vi "HEWH Gather Test Data.vi"(0 "MW100":refnum<visa-resource-name>="MW100", 1 "Core HEWH Data Station A":T2={"Scan Rate Adjust"=0.0, "Draw Count"=0, "Test Patten Setup"={"Total Gallons Schedule"=[], "PRAT/RLT Sequence"=[{"Sequence #"=1.0, "Cycles"=35, "Mode Setting"="", "Flow Rate (GPM)"=0.0, "Temperature (F)"=0.0, "Reset Timer"=FALSE, "Use Temp Decline Method"=FALSE, "Terminate Condition"=enum."C1-Terminate Draw @ Gallon Mark", "Condition Value #1"=0.0, "UE"=FALSE, "LE"=FALSE, "Comp"=FALSE, "Fan"=FALSE, "Test End Time (Sec)"=0.0, "Purge Until Cutout"=FALSE, "Start Conditions"=enum."Heat Source Cutout", "Condition Value #2"=0.0, "Remove Power"=FALSE, "Time"=0.0, "Check Special Cond."=enum."SC1-Do Nothing", "Condition#"=enum."C1", "Draw Flags"=enum."N/A", "Data Processing Delay (FHD 15sec, UEF 5 Sec)"=0.0, "Test Complete"=FALSE}, {"Sequence #"=2.0, "Cycles"=15, "Mode Setting"="", "Flow Rate (GPM)"=0.0, "Temperature (F)"=0.0, "Reset Timer"=FALSE, "Use Temp Decline Method"=FALSE, "Terminate Condition"=enum."C1-Terminate Draw @ Gallon Mark", "Condition Value #1"=0.0, "UE"=FALSE, "LE"=FALSE, "Comp"=FALSE, "Fan"=FALSE, "Test End Time (Sec)"=0.0, "Purge Until Cutout"=FALSE, "Start Conditions"=enum."Heat Source Cutout", "Condition Value #2"=0.0, "Remove Power"=FALSE, "Time"=0.0, "Check Special Cond."=enum."SC1-Do Nothing", "Condition#"=enum."C1", "Draw Flags"=enum."N/A", "Data Processing Delay (FHD 15sec, UEF 5 Sec)"=0.0, "Test Complete"=FALSE}, {"Sequence #"=3.0, "Cycles"=35, "Mode Setting"="", "Flow Rate (GPM)"=0.0, "Temperature (F)"=0.0, "Reset Timer"=FALSE, "Use Temp Decline Method"=FALSE, "Terminate Condition"=enum."C1-Terminate Draw @ Gallon Mark", "Condition Value #1"=0.0, "UE"=FALSE, "LE"=FALSE, "Comp"=FALSE, "Fan"=FALSE, "Test End Time (Sec)"=0.0, "Purge Until Cutout"=FALSE, "Start Conditions"=enum."Heat Source Cutout", "Condition Value #2"=0.0, "Remove Power"=FALSE, "Time"=0.0, "Check Special Cond."=enum."SC1-Do Nothing", "Condition#"=enum."C1", "Draw Flags"=enum."N/A", "Data Processing Delay (FHD 15sec, UEF 5 Sec)"=0.0, "Test Complete"=FALSE}, {"Sequence #"=4.0, "Cycles"=15, "Mode Setting"="", "Flow Rate (GPM)"=0.0, "Temperature (F)"=0.0, "Reset Timer"=FALSE, "Use Temp Decline Method"=FALSE, "Terminate Condition"=enum."C1-Terminate Draw @ Gallon Mark", "Condition Value #1"=0.0, "UE"=FALSE, "LE"=FALSE, "Comp"=FALSE, "Fan"=FALSE, "Test End Time (Sec)"=0.0, "Purge Until Cutout"=FALSE, "Start Conditions"=enum."Heat Source Cutout", "Condition Value #2"=0.0, "Remove Power"=FALSE, "Time"=0.0, "Check Special Cond."=enum."SC1-Do Nothing", "Condition#"=enum."C1", "Draw Flags"=enum."N/A", "Data Processing Delay (FHD 15sec, UEF 5 Sec)"=0.0, "Test Complete"=FALSE}, {"Sequence #"=5.0, "Cycles"=35, "Mode Setting"="", "Flow Rate (GPM)"=0.0, "Temperature (F)"=0.0, "Reset Timer"=FALSE, "Use Temp Decline Method"=FALSE, "Terminate Condition"=enum."C1-Terminate Draw @ Gallon Mark", "Condition Value #1"=0.0, "UE"=FALSE, "LE"=FALSE, "Comp"=FALSE, "Fan"=FALSE, "Test End Time (Sec)"=0.0, "Purge Until Cutout"=FALSE, "Start Conditions"=enum."Heat Source Cutout", "Condition Value #2"=0.0, "Remove Power"=FALSE, "Time"=0.0, "Check Special Cond."=enum."SC1-Do Nothing", "Condition#"=enum."C1", "Draw Flags"=enum."N/A", "Data Processing Delay (FHD 15sec, UEF 5 Sec)"=0.0, "Test Complete"=FALSE}, {"Sequence #"=6.0, "Cycles"=15, "Mode Setting"="", "Flow Rate (GPM)"=0.0, "Temperature (F)"=0.0, "Reset Timer"=FALSE, "Use Temp Decline Method"=FALSE, "Terminate Condition"=enum."C1-Terminate Draw @ Gallon Mark", "Condition Value #1"=0.0, "UE"=FALSE, "LE"=FALSE, "Comp"=FALSE, "Fan"=FALSE, "Test End Time (Sec)"=0.0, "Purge Until Cutout"=FALSE, "Start Conditions"=enum."Heat Source Cutout", "Condition Value #2"=0.0, "Remove Power"=FALSE, "Time"=0.0, "Check Special Cond."=enum."SC1-Do Nothing", "Condition#"=enum."C1", "Draw Flags"=enum."N/A", "Data Processing Delay (FHD 15sec, UEF 5 Sec)"=0.0, "Test Complete"=FALSE}, {"Sequence #"=7.0, "Cycles"=35, "Mode Setting"="", "Flow Rate (GPM)"=0.0, "Temperature (F)"=0.0, "Reset Timer"=FALSE, "Use Temp Decline Method"=FALSE, "Terminate Condition"=enum."C1-Terminate Draw @ Gallon Mark", "Condition Value #1"=0.0, "UE"=FALSE, "LE"=FALSE, "Comp"=FALSE, "Fan"=FALSE, "Test End Time (Sec)"=0.0, "Purge Until Cutout"=FALSE, "Start Conditions"=enum."Heat Source Cutout", "Condition Value #2"=0.0, "Remove Power"=FALSE, "Time"=0.0, "Check Special Cond."=enum."SC1-Do Nothing", "Condition#"=enum."C1", "Draw Flags"=enum."N/A", "Data Processing Delay (FHD 15sec, UEF 5 Sec)"=0.0, "Test Complete"=FALSE}, {"Sequence #"=8.0, "Cycles"=15, "Mode Setting"="", "Flow Rate (GPM)"=0.0, "Temperature (F)"=0.0, "Reset Timer"=FALSE, "Use Temp Decline Method"=FALSE, "Terminate Condition"=enum."C1-Terminate Draw @ Gallon Mark", "Condition Value #1"=0.0, "UE"=FALSE, "LE"=FALSE, "Comp"=FALSE, "Fan"=FALSE, "Test End Time (Sec)"=0.0, "Purge Until Cutout"=FALSE, "Start Conditions"=enum."Heat Source Cutout", "Condition Value #2"=0.0, "Remove Power"=FALSE, "Time"=0.0, "Check Special Cond."=enum."SC1-Do Nothing", "Condition#"=enum."C1", "Draw Flags"=enum."N/A", "Data Processing Delay (FHD 15sec, UEF 5 Sec)"=0.0, "Test Complete"=FALSE}], "Current Sequence Index"=0}, "HEWH Specific DAQ"={"HEWH Data"={"HEWH Standard"={"Voltage (Volts)"=0.0, "Current (Amps)"=0.0, "Power (Watts)"=0.0, "WattHours (Wh)"=0.0, "TC Tree (AVG)"=0.0, "Flow Rate (GPM)"=0.0, "Gallons (Gal)"=0.0, "RTD Out (Deg F)"=0.0, "RTD In (Deg F)"=0.0, "RTD Amb (Deg F)"=0.0, "TC Down"=0.0, "UE Event Lead"=0, "LE Event Lead"=0, "TC Tree Array"=[]}, "PRAT"={"Power (Watts) A"=4192.0, "Power (Watts) B"=4192.0, "Power (Watts) C"=4192.0, "Power (Watts) D"=4192.0, "TC1"=0.0, "TC2"=0.0, "TC3"=0.0, "TC4"=0.0, "WattHours (Wh) A"=4192.0, "WattHours (Wh) B"=4192.0, "WattHours (Wh) C"=4192.0, "WattHours (Wh) D"=4192.0, "Ambient"=0.0, "Extra Temp"=0.0}, "Additional Power Data"={"Vthd"=236.2, "Frequency (Hz)"=236.2, "Apparent Power (VA)"=236.2, "Power Factor"=236.2, "Current Crest Factor"=236.2, "Voltage Crest Factor"=236.2, "Integration Time (sec)"=236.2}}, "Flow Valve % Open"=0.0, "Power State"={"UE"=FALSE, "LE"=FALSE, "COMP"=FALSE, "FANS"=FALSE}, "Power Analyzer"=enum."APLUS", "Flow Valve uA Output"=0, "Gallons Start (Gal)"=0.0}, "Test Output Data"={"PreDraw Data Table"=[], "Data Table"=[], "MW100 TC Headers"=[]}, "Calc and Calibration"={"Mean SD Var Max Min Array"=[], "Draw Statistics (DBL)"=[], "Calibration Coefficients DBL"=[], "Start Gallons"=0.0, "Starting Temp Decline"=0.0, "K-Factor (Intellifaucet)"=0.0, "All Draw Stats"=[], "RTD Terminate Value"=0.0}, "Current Draw Time"=0.0, "LV Program"=enum."HEWH", "Station ID"=enum."A", "Current Cond"=enum."N/A", "Test Complete"=FALSE} {"Test Patten Setup"."PRAT/RLT Sequence"."Time" format="%<%H:%M:%S>t"; "Test Patten Setup"."Total Gallons Schedule" format="%.2f"}, 2 "GEA2?":bool, 4 "Yokogawa WT210":refnum<visa-resource-name>, 5 "error in (no error)":errorcluster, 6 "Laurel IP Address":string, 9 "Draw Count":i32, 11 "Use Emerson 5700?":bool) -> (14 "MW100 Output":refnum<visa-resource-name>, 15 "Core HEWH Data Station A":T2={"Scan Rate Adjust"=0.0, "Draw Count"=0, "Test Patten Setup"={"Total Gallons Schedule"=[], "PRAT/RLT Sequence"=[{"Sequence #"=1.0, "Cycles"=35, "Mode Setting"="", "Flow Rate (GPM)"=0.0, "Temperature (F)"=0.0, "Reset Timer"=FALSE, "Use Temp Decline Method"=FALSE, "Terminate Condition"=enum."C1-Terminate Draw @ Gallon Mark", "Condition Value #1"=0.0, "UE"=FALSE, "LE"=FALSE, "Comp"=FALSE, "Fan"=FALSE, "Test End Time (Sec)"=0.0, "Purge Until Cutout"=FALSE, "Start Conditions"=enum."Heat Source Cutout", "Condition Value #2"=0.0, "Remove Power"=FALSE, "Time"=0.0, "Check Special Cond."=enum."SC1-Do Nothing", "Condition#"=enum."C1", "Draw Flags"=enum."N/A", "Data Processing Delay (FHD 15sec, UEF 5 Sec)"=0.0, "Test Complete"=FALSE}, {"Sequence #"=2.0, "Cycles"=15, "Mode Setting"="", "Flow Rate (GPM)"=0.0, "Temperature (F)"=0.0, "Reset Timer"=FALSE, "Use Temp Decline Method"=FALSE, "Terminate Condition"=enum."C1-Terminate Draw @ Gallon Mark", "Condition Value #1"=0.0, "UE"=FALSE, "LE"=FALSE, "Comp"=FALSE, "Fan"=FALSE, "Test End Time (Sec)"=0.0, "Purge Until Cutout"=FALSE, "Start Conditions"=enum."Heat Source Cutout", "Condition Value #2"=0.0, "Remove Power"=FALSE, "Time"=0.0, "Check Special Cond."=enum."SC1-Do Nothing", "Condition#"=enum."C1", "Draw Flags"=enum."N/A", "Data Processing Delay (FHD 15sec, UEF 5 Sec)"=0.0, "Test Complete"=FALSE}, {"Sequence #"=3.0, "Cycles"=35, "Mode Setting"="", "Flow Rate (GPM)"=0.0, "Temperature (F)"=0.0, "Reset Timer"=FALSE, "Use Temp Decline Method"=FALSE, "Terminate Condition"=enum."C1-Terminate Draw @ Gallon Mark", "Condition Value #1"=0.0, "UE"=FALSE, "LE"=FALSE, "Comp"=FALSE, "Fan"=FALSE, "Test End Time (Sec)"=0.0, "Purge Until Cutout"=FALSE, "Start Conditions"=enum."Heat Source Cutout", "Condition Value #2"=0.0, "Remove Power"=FALSE, "Time"=0.0, "Check Special Cond."=enum."SC1-Do Nothing", "Condition#"=enum."C1", "Draw Flags"=enum."N/A", "Data Processing Delay (FHD 15sec, UEF 5 Sec)"=0.0, "Test Complete"=FALSE}, {"Sequence #"=4.0, "Cycles"=15, "Mode Setting"="", "Flow Rate (GPM)"=0.0, "Temperature (F)"=0.0, "Reset Timer"=FALSE, "Use Temp Decline Method"=FALSE, "Terminate Condition"=enum."C1-Terminate Draw @ Gallon Mark", "Condition Value #1"=0.0, "UE"=FALSE, "LE"=FALSE, "Comp"=FALSE, "Fan"=FALSE, "Test End Time (Sec)"=0.0, "Purge Until Cutout"=FALSE, "Start Conditions"=enum."Heat Source Cutout", "Condition Value #2"=0.0, "Remove Power"=FALSE, "Time"=0.0, "Check Special Cond."=enum."SC1-Do Nothing", "Condition#"=enum."C1", "Draw Flags"=enum."N/A", "Data Processing Delay (FHD 15sec, UEF 5 Sec)"=0.0, "Test Complete"=FALSE}, {"Sequence #"=5.0, "Cycles"=35, "Mode Setting"="", "Flow Rate (GPM)"=0.0, "Temperature (F)"=0.0, "Reset Timer"=FALSE, "Use Temp Decline Method"=FALSE, "Terminate Condition"=enum."C1-Terminate Draw @ Gallon Mark", "Condition Value #1"=0.0, "UE"=FALSE, "LE"=FALSE, "Comp"=FALSE, "Fan"=FALSE, "Test End Time (Sec)"=0.0, "Purge Until Cutout"=FALSE, "Start Conditions"=enum."Heat Source Cutout", "Condition Value #2"=0.0, "Remove Power"=FALSE, "Time"=0.0, "Check Special Cond."=enum."SC1-Do Nothing", "Condition#"=enum."C1", "Draw Flags"=enum."N/A", "Data Processing Delay (FHD 15sec, UEF 5 Sec)"=0.0, "Test Complete"=FALSE}, {"Sequence #"=6.0, "Cycles"=15, "Mode Setting"="", "Flow Rate (GPM)"=0.0, "Temperature (F)"=0.0, "Reset Timer"=FALSE, "Use Temp Decline Method"=FALSE, "Terminate Condition"=enum."C1-Terminate Draw @ Gallon Mark", "Condition Value #1"=0.0, "UE"=FALSE, "LE"=FALSE, "Comp"=FALSE, "Fan"=FALSE, "Test End Time (Sec)"=0.0, "Purge Until Cutout"=FALSE, "Start Conditions"=enum."Heat Source Cutout", "Condition Value #2"=0.0, "Remove Power"=FALSE, "Time"=0.0, "Check Special Cond."=enum."SC1-Do Nothing", "Condition#"=enum."C1", "Draw Flags"=enum."N/A", "Data Processing Delay (FHD 15sec, UEF 5 Sec)"=0.0, "Test Complete"=FALSE}, {"Sequence #"=7.0, "Cycles"=35, "Mode Setting"="", "Flow Rate (GPM)"=0.0, "Temperature (F)"=0.0, "Reset Timer"=FALSE, "Use Temp Decline Method"=FALSE, "Terminate Condition"=enum."C1-Terminate Draw @ Gallon Mark", "Condition Value #1"=0.0, "UE"=FALSE, "LE"=FALSE, "Comp"=FALSE, "Fan"=FALSE, "Test End Time (Sec)"=0.0, "Purge Until Cutout"=FALSE, "Start Conditions"=enum."Heat Source Cutout", "Condition Value #2"=0.0, "Remove Power"=FALSE, "Time"=0.0, "Check Special Cond."=enum."SC1-Do Nothing", "Condition#"=enum."C1", "Draw Flags"=enum."N/A", "Data Processing Delay (FHD 15sec, UEF 5 Sec)"=0.0, "Test Complete"=FALSE}, {"Sequence #"=8.0, "Cycles"=15, "Mode Setting"="", "Flow Rate (GPM)"=0.0, "Temperature (F)"=0.0, "Reset Timer"=FALSE, "Use Temp Decline Method"=FALSE, "Terminate Condition"=enum."C1-Terminate Draw @ Gallon Mark", "Condition Value #1"=0.0, "UE"=FALSE, "LE"=FALSE, "Comp"=FALSE, "Fan"=FALSE, "Test End Time (Sec)"=0.0, "Purge Until Cutout"=FALSE, "Start Conditions"=enum."Heat Source Cutout", "Condition Value #2"=0.0, "Remove Power"=FALSE, "Time"=0.0, "Check Special Cond."=enum."SC1-Do Nothing", "Condition#"=enum."C1", "Draw Flags"=enum."N/A", "Data Processing Delay (FHD 15sec, UEF 5 Sec)"=0.0, "Test Complete"=FALSE}], "Current Sequence Index"=0}, "HEWH Specific DAQ"={"HEWH Data"={"HEWH Standard"={"Voltage (Volts)"=0.0, "Current (Amps)"=0.0, "Power (Watts)"=0.0, "WattHours (Wh)"=0.0, "TC Tree (AVG)"=0.0, "Flow Rate (GPM)"=0.0, "Gallons (Gal)"=0.0, "RTD Out (Deg F)"=0.0, "RTD In (Deg F)"=0.0, "RTD Amb (Deg F)"=0.0, "TC Down"=0.0, "UE Event Lead"=0, "LE Event Lead"=0, "TC Tree Array"=[]}, "PRAT"={"Power (Watts) A"=4192.0, "Power (Watts) B"=4192.0, "Power (Watts) C"=4192.0, "Power (Watts) D"=4192.0, "TC1"=0.0, "TC2"=0.0, "TC3"=0.0, "TC4"=0.0, "WattHours (Wh) A"=4192.0, "WattHours (Wh) B"=4192.0, "WattHours (Wh) C"=4192.0, "WattHours (Wh) D"=4192.0, "Ambient"=0.0, "Extra Temp"=0.0}, "Additional Power Data"={"Vthd"=236.2, "Frequency (Hz)"=236.2, "Apparent Power (VA)"=236.2, "Power Factor"=236.2, "Current Crest Factor"=236.2, "Voltage Crest Factor"=236.2, "Integration Time (sec)"=236.2}}, "Flow Valve % Open"=0.0, "Power State"={"UE"=FALSE, "LE"=FALSE, "COMP"=FALSE, "FANS"=FALSE}, "Power Analyzer"=enum."APLUS", "Flow Valve uA Output"=0, "Gallons Start (Gal)"=0.0}, "Test Output Data"={"PreDraw Data Table"=[], "Data Table"=[], "MW100 TC Headers"=[]}, "Calc and Calibration"={"Mean SD Var Max Min Array"=[], "Draw Statistics (DBL)"=[], "Calibration Coefficients DBL"=[], "Start Gallons"=0.0, "Starting Temp Decline"=0.0, "K-Factor (Intellifaucet)"=0.0, "All Draw Stats"=[], "RTD Terminate Value"=0.0}, "Current Draw Time"=0.0, "LV Program"=enum."HEWH", "Station ID"=enum."A", "Current Cond"=enum."N/A", "Test Complete"=FALSE} {"Test Patten Setup"."PRAT/RLT Sequence"."Time" format="%<%H:%M:%S>t"; "Test Patten Setup"."Total Gallons Schedule" format="%.2f"}, 16 "Display Message":string, 17 "Emerson Flow Meter Data Output":T1, 18 "MW100 Full Data":string[][](array[string]), 19 "error out":errorcluster={"status"=TRUE, "code"=-1073807346, "source"="VISA Read in Gather Test Data.vi"})   [LabVIEW 2016]
uses:
  Type Definitions/HEWH Output Information.ctl
  Type Definitions/HEWH Draw Pattern Setup.ctl
  Type Definitions/PRAT Test.ctl
  Utility/Save File/File Setup (Public)/Type Definition/Save File HEWH Heating Control Mode.ctl
  Support VIs/Draw Water Specific/Type Definitions/Terminate Draw Conditions.ctl
  Type Definitions/HEWH Start Conditions.ctl
  Support VIs/Draw Water Specific/Type Definitions/Check Special Condtions.ctl
  Support VIs/Draw Water Specific/Type Definitions/HEWH Special Condition Check.ctl
  Type Definitions/HEWH Draw Flag ENUM.ctl
  Type Definitions/HEWH Specific DAQ.ctl
  Type Definitions/HEWH Power Data.ctl
  Type Definitions/HEWH Power Elements.ctl
  Utility/Type Definitions/UTILITY Power Analyzer.ctl
  Type Definitions/HEWH Calc and Calibration.ctl
  Utility/Save File/File Setup (Public)/Type Definition/Save File DOE LabView Program.ctl
  MW100/Type Definitions/Station ID Selector.ctl
  Drivers/Emerson 5700 Transmitter/Type Definitions/Emerson 5700 Data.ctl
  Utility/Type Definitions/UTILITY Power Data.ctl
  Drivers/Laurel Meter/Type Definitions/Laurel Serial Commands.ctl
  Type Definitions/HEWH MW100 Data Cluster.ctl
  Utility/Save File/File Setup.lvlib
panel:
  # "Draw Pattern Setup (24 Hour)"
  # "Draw Pattern Setup (24 Hour)"
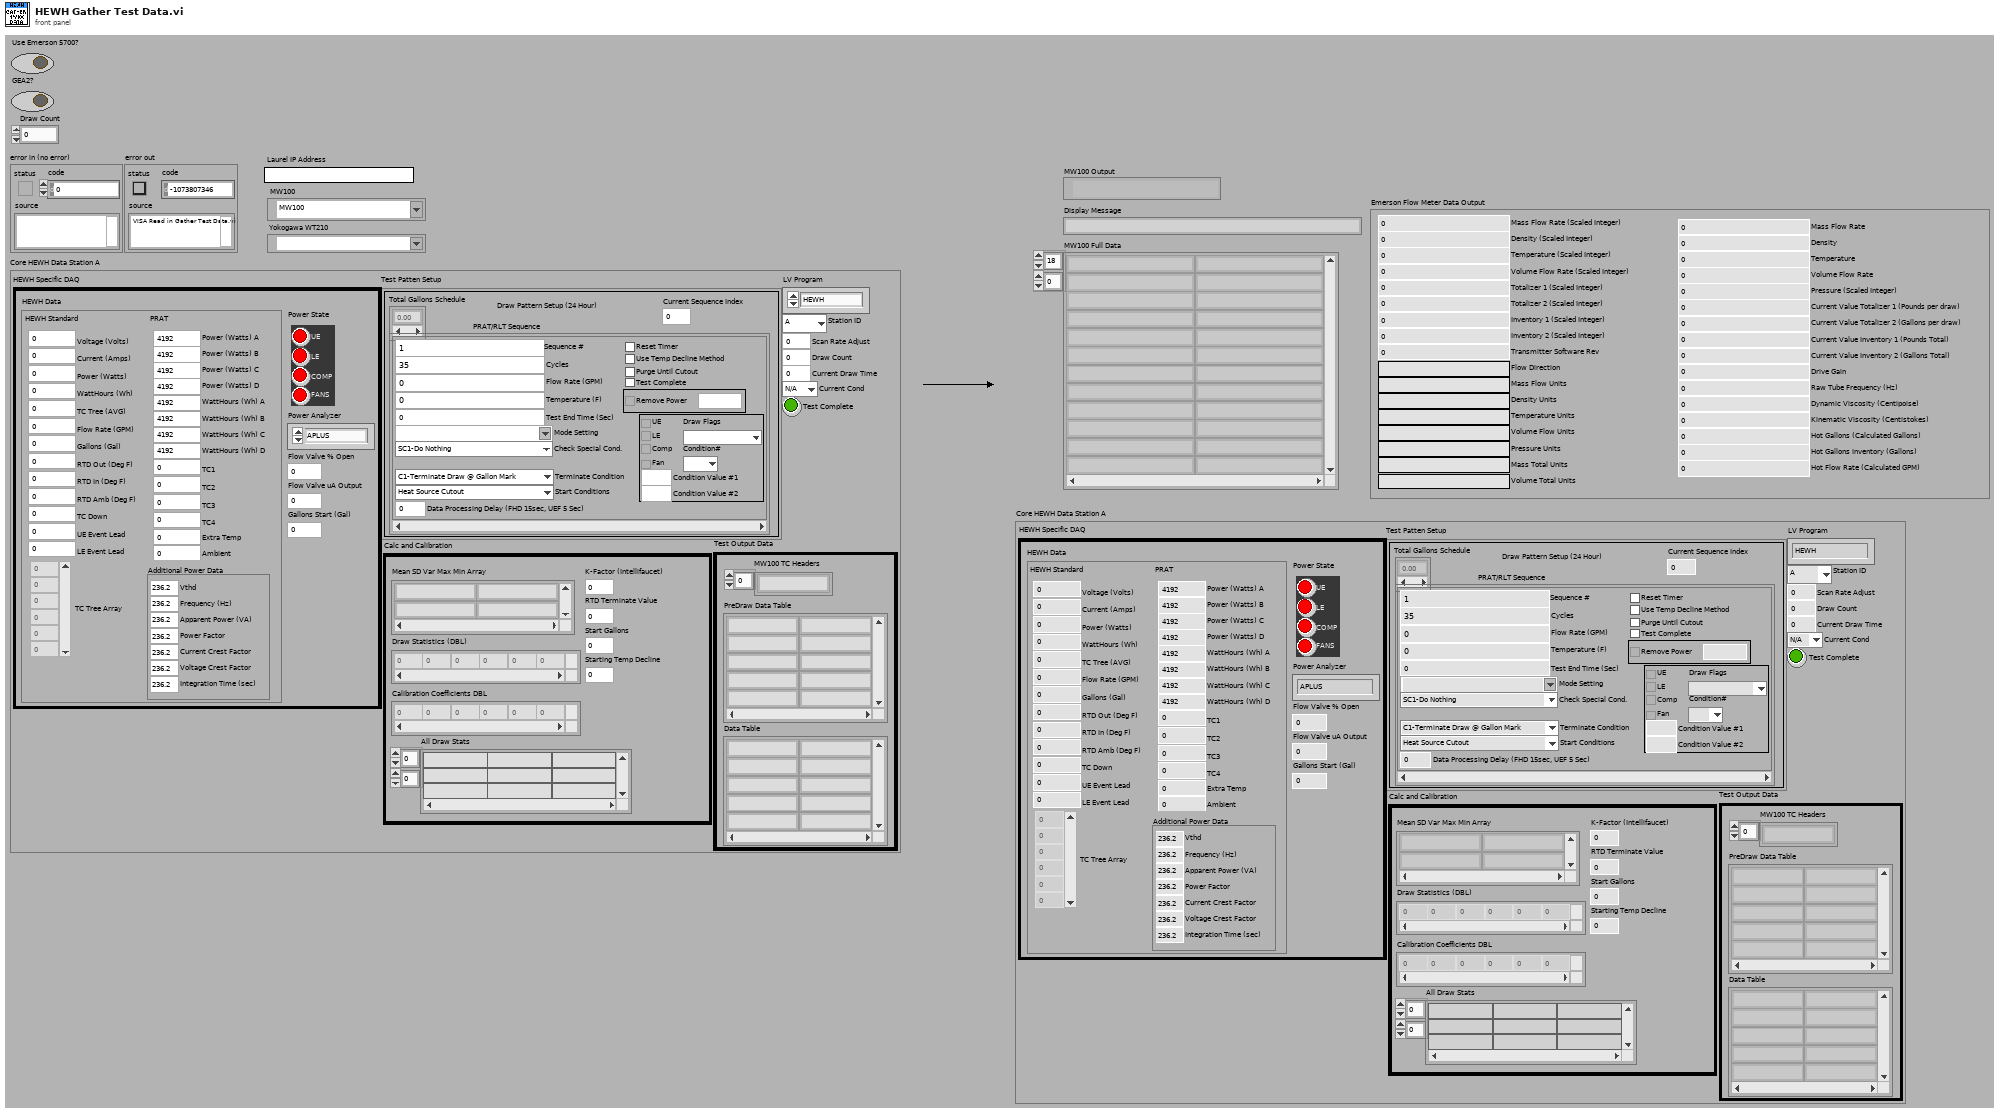
[diagram p1: front panel]
types:
  T1 = typedef "Emerson 5700 Data.ctl" = cluster{"Mass Flow Rate (Scaled Integer)":u16, "Density (Scaled Integer)":u16, "Temperature (Scaled Integer)":u16, "Volume Flow Rate (Scaled Integer)":u16, "Totalizer 1 (Scaled Integer)":u16, "Totalizer 2 (Scaled Integer)":u16, "Transmitter Software Rev":u16, "Flow Direction":string, "Mass Flow Units":string, "Density Units":string, "Temperature Units":string, "Volume Flow Units":string, "Pressure Units":string, "Mass Total Units":string, "Volume Total Units":string, "Inventory 1 (Scaled Integer)":u16, "Inventory 2 (Scaled Integer)":u16, "Mass Flow Rate":dbl, "Density":dbl, "Temperature":dbl, "Volume Flow Rate":dbl, "Pressure (Scaled Integer)":u16, "Current Value Totalizer 1 (Pounds per draw)":dbl, "Current Value Totalizer 2 (Gallons per draw)":dbl, "Current Value Inventory 1 (Pounds Total)":dbl, "Current Value Inventory 2 (Gallons Total)":dbl, "Drive Gain":dbl, "Raw Tube Frequency (Hz)":dbl, "Dynamic Viscosity (Centipoise)":dbl, "Kinematic Viscosity (Centistokes)":dbl, "Hot Gallons (Calculated Gallons)":dbl, "Hot Flow Rate (Calculated GPM)":dbl, "Hot Gallons Inventory (Gallons)":dbl}
  T2 = typedef "HEWH Output Information.ctl" = cluster{"Scan Rate Adjust":dbl, "Draw Count":i32, "Test Patten Setup":T3, "HEWH Specific DAQ":T11, "Test Output Data":cluster{"PreDraw Data Table":string[][], "Data Table":string[][], "MW100 TC Headers":string[]}, "Calc and Calibration":T15, "Current Draw Time":dbl, "LV Program":T16, "Station ID":T17, "Current Cond":T9, "Test Complete":bool}
  T3 = typedef "HEWH Draw Pattern Setup.ctl" = cluster{"Total Gallons Schedule":dbl[], "PRAT/RLT Sequence":T4[], "Current Sequence Index":i32}
  T4 = typedef "PRAT Test.ctl" = cluster{"Sequence #":dbl, "Cycles":i32, "Mode Setting":T5, "Flow Rate (GPM)":dbl, "Temperature (F)":dbl, "Reset Timer":bool, "Use Temp Decline Method":bool, "Terminate Condition":T6, "Condition Value #1":dbl, "UE":bool, "LE":bool, "Comp":bool, "Fan":bool, "Test End Time (Sec)":dbl, "Purge Until Cutout":bool, "Start Conditions":T7, "Condition Value #2":dbl, "Remove Power":bool, "Time":dbl, "Check Special Cond.":T8, "Condition#":T9, "Draw Flags":T10, "Data Processing Delay (FHD 15sec, UEF 5 Sec)":dbl, "Test Complete":bool}
  T5 = typedef "File Setup.lvlib/Save File HEWH Heating Control Mode.ctl" = string
  T6 = typedef "Terminate Draw Conditions.ctl" = enum16{"C1-Terminate Draw @ Gallon Mark", "C2-Special Last Draw (HU Test)", "C3-RTD Out <=", "C4-Mean Tank Temp <=", "C5-Decrease RTD Out (Deg F)", "C6-Time (Seconds)", "C7-Until Any Heat Source", "C8-Specific Heat Source", "C9-Do Nothing"}
  T7 = typedef "HEWH Start Conditions.ctl" = enum16{"Heat Source Cutout", "At Time (Seconds)", "Every X (Seconds)", "T2 >= X° Below Setpoint", "Seconds From Complete", "Wait for LE & Comp Cutout", "Wait for Comp Cutout", "Wait for LE Cutout", "Wait for UE Cutout"}
  T8 = typedef "Check Special Condtions.ctl" = enum16{"SC1-Do Nothing", "SC2-Check Heat Source (On-C2/Off-C1)", "SC3-Check Skip Condition", "SC4-Check Heat Source ON/Fail"}
  T9 = typedef "HEWH Special Condition Check.ctl" = enum16{"N/A", "C1", "C2", "Reset/Fail", "Skip Draw Sequence"}
  T10 = typedef "HEWH Draw Flag ENUM.ctl" = enum16{"N/A", "None(0)", "Sml(1)", "Med(2)", "SmlMed(3)", "Lrg(4)", "SmlLrg(5)", "MedLrg(6)", "SmlMedLrg(7)"}
  T11 = typedef "HEWH Specific DAQ.ctl" = cluster{"HEWH Data":T12, "Flow Valve % Open":dbl, "Power State":T13, "Power Analyzer":T14, "Flow Valve uA Output":i32, "Gallons Start (Gal)":dbl}
  T12 = typedef "HEWH Power Data.ctl" = cluster{"HEWH Standard":cluster{"Voltage (Volts)":dbl, "Current (Amps)":dbl, "Power (Watts)":dbl, "WattHours (Wh)":dbl, "TC Tree (AVG)":dbl, "Flow Rate (GPM)":dbl, "Gallons (Gal)":dbl, "RTD Out (Deg F)":dbl, "RTD In (Deg F)":dbl, "RTD Amb (Deg F)":dbl, "TC Down":dbl, "UE Event Lead":i32, "LE Event Lead":i32, "TC Tree Array":dbl[]}, "PRAT":cluster{"Power (Watts) A":dbl, "Power (Watts) B":dbl, "Power (Watts) C":dbl, "Power (Watts) D":dbl, "TC1":dbl, "TC2":dbl, "TC3":dbl, "TC4":dbl, "WattHours (Wh) A":dbl, "WattHours (Wh) B":dbl, "WattHours (Wh) C":dbl, "WattHours (Wh) D":dbl, "Ambient":dbl, "Extra Temp":dbl}, "Additional Power Data":cluster{"Vthd":dbl, "Frequency (Hz)":dbl, "Apparent Power (VA)":dbl, "Power Factor":dbl, "Current Crest Factor":dbl, "Voltage Crest Factor":dbl, "Integration Time (sec)":dbl}}
  T13 = typedef "HEWH Power Elements.ctl" = cluster{"UE":bool, "LE":bool, "COMP":bool, "FANS":bool}
  T14 = typedef "UTILITY Power Analyzer.ctl" = enum16{"", "APLUS", "WT210", "WT500", "WT300", "OSI", "Debug", "WT230", "WT300_1", "WT300_2"}
  T15 = typedef "HEWH Calc and Calibration.ctl" = cluster{"Mean SD Var Max Min Array":string[][], "Draw Statistics (DBL)":dbl[][], "Calibration Coefficients DBL":dbl[][], "Start Gallons":dbl, "Starting Temp Decline":dbl, "K-Factor (Intellifaucet)":dbl, "All Draw Stats":string[][], "RTD Terminate Value":dbl}
  T16 = typedef "File Setup.lvlib/Save File DOE LabView Program.ctl" = enum16{"No Name Found", "DOE Stand", "Dishwasher Kitchen", "Portable Stand", "HEWH", "Dryer", "Dryer WILT", "HCC", "PRAT", "HEWH RLT", "Refrigeration"}
  T17 = typedef "Station ID Selector.ctl" = enum16{"", "A", "B", "C", "D", "Global"}
  T18 = typedef "Laurel Serial Commands.ctl" = string
  T19 = typedef "UTILITY Power Data.ctl" = cluster{"Current (A):Element 1":dbl, "Current (A):Element 2":dbl, "Power (W):Sigma":dbl, "Watt Hours (Wh):Sigma":dbl, "Voltage (V):Element 2":dbl, "Voltage (V):Element 1":dbl, "Current Crest Factor:Element 1":dbl, "Current Crest Factor:Element 2":dbl, "Voltage Harmonic (%):Element 1":dbl, "Voltage Harmonic (%):Element 2":dbl, "Voltage Crest Factor:Element 1":dbl, "Voltage Crest Factor:Element 2":dbl, "Time:Element 1":dbl, "Frequency (Hz):Element 1":dbl, "Apparent Power (VA):Element 1":dbl, "Apparent Power (VA):Element 2":dbl, "Power Factor:Element 1":dbl, "Power Factor:Element 2":dbl, "Max Watt Hours":dbl, "Voltage (V):Element 2 Avg":dbl, "Voltage (V):Element 1 Avg":dbl}
  T20 = typedef "HEWH MW100 Data Cluster.ctl" = cluster{"T1":dbl, "T2":dbl, "T3":dbl, "T4":dbl, "T5":dbl, "T6":dbl, "T7":dbl, "T8":dbl, "T9":dbl, "T10":dbl, "TC Tree Average":dbl, "TC DOWN":dbl, "RTD IN":dbl, "RTD OUT":dbl, "RTD AMB":dbl, "Voltage (0-300VAC)":dbl, "Current":dbl, "Watts (Raw Voltage OSI)":dbl, "Voltage (OSI) 0-10V=300VAC":dbl, "Watt Hour Ticker":dbl, "Watt Hours (OSI)":dbl, "Flow Meter Voltage Output":dbl, "Totalized Flow (Linear Link GAL) - Calculated":dbl, "Unfiltered Flow (Linear Link)":dbl, "Flow Rate (Linear Link GPM) - Calculated":dbl, "Pressure - HI 1":dbl, "Pressure - HI 2":dbl, "Pressure - Low":dbl, "Pres_PIN":dbl, "UE-State(1/0 on off)":dbl, "LE-State(1/0 on off)":dbl, "CALC1":dbl, "CALC2":dbl, "CALC3":dbl, "CALC4":dbl, "CALC5":dbl, "CALC6 - 10 Point Moving Avg":dbl, "NA2":dbl, "NA3":dbl}
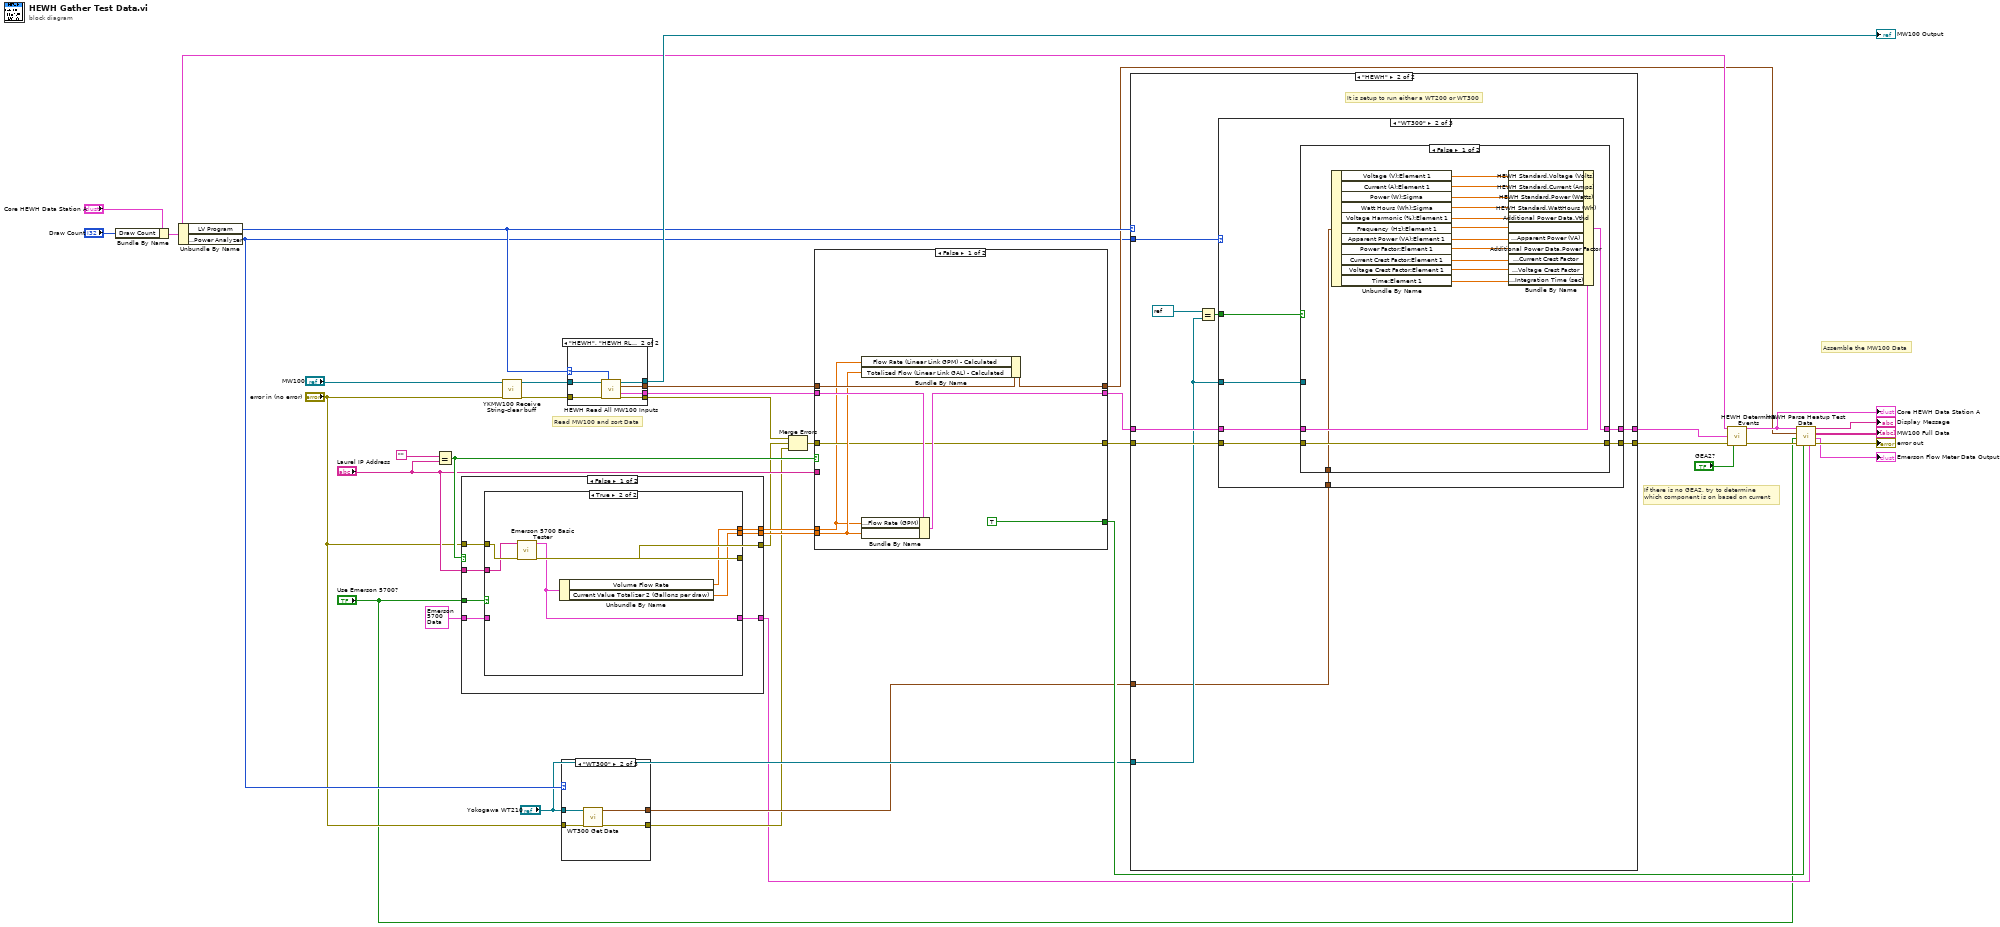
[diagram p0: block diagram]
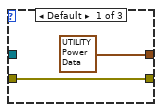
[diagram p2: hidden frame]
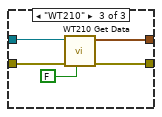
[diagram p3: hidden frame]
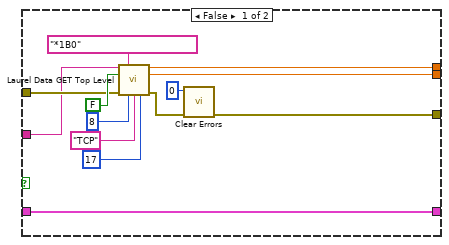
[diagram p4: hidden frame]
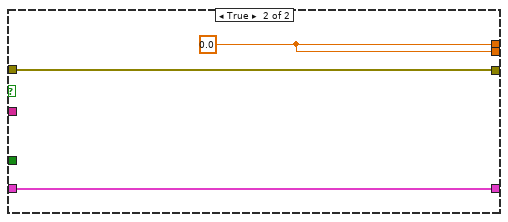
[diagram p5: hidden frame]
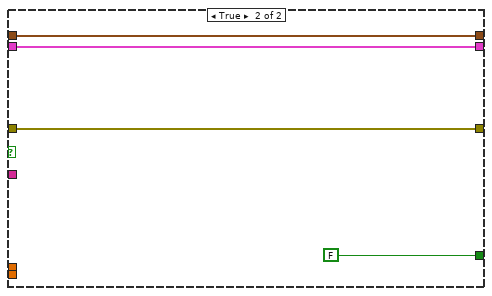
[diagram p6: hidden frame]
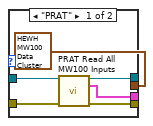
[diagram p7: hidden frame]
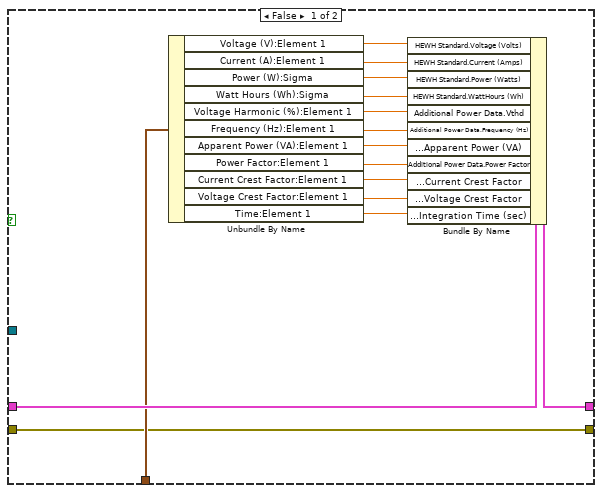
[diagram p12: hidden frame]
diagram:
  # "Assemble the MW100 Data"
  # "If there is no GEA2, try to determine \nwhich component is on based on current"
  # "Read MW100 and sort Data"
  n1 = Bundle By Name(cluster="Core HEWH Data Station A", "Draw Count"="Draw Count") -> (w28:T2)
  n2 = Unbundle By Name(w28) -> ("LV Program"=w25:T16, "HEWH Specific DAQ.Power Analyzer"=w9:T14)
  n3 = Equal?(x="", y="Laurel IP Address") -> (x = y?=w16:bool)
  n4 = case shown="False" w16 {
    tunnel: "Laurel IP Address" -> [w46 _]
    tunnel: "error in (no error)" -> [w47 w69]
    tunnel: [w43 w69] -> w11
    tunnel: [w45 w68] -> w14
    tunnel: [w44 w68] -> w13
    tunnel: "Use Emerson 5700?" -> [w42 _]
    tunnel: [w41 w67] -> w4
    tunnel: T1 {"Mass Flow Rate (Scaled Integer)"=0, "Density (Scaled Integer)"=0, "Temperature (Scaled Integer)"=0, "Volume Flow Rate (Scaled Integer)"=0, "Totalizer 1 (Scaled Integer)"=0, "Totalizer 2 (Scaled Integer)"=0, "Transmitter Software Rev"=0, "Flow Direction"="", "Mass Flow Units"="", "Density Units"="", "Temperature Units"="", "Volume Flow Units"="", "Pressure Units"="", "Mass Total Units"="", "Volume Total Units"="", "Inventory 1 (Scaled Integer)"=0, "Inventory 2 (Scaled Integer)"=0, "Mass Flow Rate"=0.0, "Density"=0.0, "Temperature"=0.0, "Volume Flow Rate"=0.0, "Pressure (Scaled Integer)"=0, "Current Value Totalizer 1 (Pounds per draw)"=0.0, "Current Value Totalizer 2 (Gallons per draw)"=0.0, "Current Value Inventory 1 (Pounds Total)"=0.0, "Current Value Inventory 2 (Gallons Total)"=0.0, "Drive Gain"=0.0, "Raw Tube Frequency (Hz)"=0.0, "Dynamic Viscosity (Centipoise)"=0.0, "Kinematic Viscosity (Centistokes)"=0.0, "Hot Gallons (Calculated Gallons)"=0.0, "Hot Flow Rate (Calculated GPM)"=0.0, "Hot Gallons Inventory (Gallons)"=0.0} ("Emerson Flow Meter Data Output") -> [w40 w67]
    frame False {
      n5 = case shown="True" w42 {
        tunnel: w47 -> [w55 w66]
        tunnel: w46 -> [w54 w64]
        tunnel: [w53 w63] -> w45
        tunnel: [w52 w62] -> w44
        tunnel: [w50 w65] -> w43
        tunnel: [w48 w61] -> w41
        tunnel: w40 -> [w48 _]
        frame False {
          n6 = call "Laurel Data GET Top Level.vi"("Laurel IP Address"=w54, "Laurel Serial Commands"=T18 "*1B0", "Use Delay"=FALSE, "error in (no error)"=w55, "byte count"=8, "Laurel Communication Type"="TCP", "All Items Byte Count (Flow Rate)"=17 ("byte count")) -> ("Flow Rate (Item 1)"=w53:dbl, "Gallons (Item 2)"=w52:dbl, "error out"=w51:errorcluster)  [unwired: 3 in, 3 out]
          n7 = call <vilib>:"Clear Errors.vi"("error in (no error)"=w51, "specific error code to clear (0: all)"=0) -> ("error out"=w50:errorcluster)  [unwired: 4 in, 1 out]
        }
        frame True {
          n8 = call "Emerson 5700 Basic Tester.vi"("Error In"=w66, "Remote IP Address"=w64) -> ("Error Out"=w65:errorcluster, "Emerson Flow Meter Data Output"=w61:T1)  [unwired: 8 in]
          n9 = Unbundle By Name(w61) -> ("Volume Flow Rate"=w63:dbl, "Current Value Totalizer 2 (Gallons per draw)"=w62:dbl)
        }
      }
    }
    frame True {
      w68 = 0.0 ("Flow Rate (Item 1)")
    }
  }
  n10 = call "YKMW100 Receive String-clear buff.vi"("VISA session"="MW100", "error in (no error)"="error in (no error)") -> ("dup VISA session"=w39:refnum<visa-resource-name>, "error out"=w38:errorcluster)  [unwired: 11 in, 1 out]
  n11 = case shown="\"WT300\"" w9 {
    tunnel: "Yokogawa WT210" -> [_ w75 w79]
    tunnel: "error in (no error)" -> [w71 w74 w78]
    tunnel: [w71 w73 w77] -> w5
    tunnel: [T19 {"Current (A):Element 1"=0.0, "Current (A):Element 2"=0.0, "Power (W):Sigma"=0.0, "Watt Hours (Wh):Sigma"=0.0, "Voltage (V):Element 2"=0.0, "Voltage (V):Element 1"=0.0, "Current Crest Factor:Element 1"=0.0, "Current Crest Factor:Element 2"=0.0, "Voltage Harmonic (%):Element 1"=0.0, "Voltage Harmonic (%):Element 2"=0.0, "Voltage Crest Factor:Element 1"=0.0, "Voltage Crest Factor:Element 2"=0.0, "Time:Element 1"=0.0, "Frequency (Hz):Element 1"=0.0, "Apparent Power (VA):Element 1"=0.0, "Apparent Power (VA):Element 2"=0.0, "Power Factor:Element 1"=0.0, "Power Factor:Element 2"=0.0, "Max Watt Hours"=0.0, "Voltage (V):Element 2 Avg"=0.0, "Voltage (V):Element 1 Avg"=0.0} ("Power Data") w72 w76] -> w6
    frame Default {
    }
    frame "WT300" {
      n12 = call "WT300 Get Data.vi"("error in (no error)"=w74, "VISA resource name"=w75) -> ("error out"=w73:errorcluster, "Power Data"=w72:T19)  [unwired: 4 in, 4 out]
    }
    frame "WT210" {
      n13 = call "WT210 Get Data.vi"("Collect Element 3 Data"=FALSE, "error in (no error)"=w78, "VISA resource name"=w79) -> ("error out"=w77:errorcluster, "Power Data"=w76:T19)  [unwired: 3 in, 4 out]
    }
  }
  n14 = case shown="\"HEWH\", \"HEWH RLT\", Default" w25 {
    selector: w25 -> [_ w87]
    tunnel: w39 -> [w86 w93]
    tunnel: w38 -> [w85 w92]
    tunnel: [T20 {"T1"=0.0, "T2"=0.0, "T3"=0.0, "T4"=0.0, "T5"=0.0, "T6"=0.0, "T7"=0.0, "T8"=0.0, "T9"=0.0, "T10"=0.0, "TC Tree Average"=0.0, "TC DOWN"=0.0, "RTD IN"=0.0, "RTD OUT"=0.0, "RTD AMB"=0.0, "Voltage (0-300VAC)"=0.0, "Current"=0.0, "Watts (Raw Voltage OSI)"=0.0, "Voltage (OSI) 0-10V=300VAC"=0.0, "Watt Hour Ticker"=0.0, "Watt Hours (OSI)"=0.0, "Flow Meter Voltage Output"=0.0, "Totalized Flow (Linear Link GAL) - Calculated"=0.0, "Unfiltered Flow (Linear Link)"=0.0, "Flow Rate (Linear Link GPM) - Calculated"=0.0, "Pressure - HI 1"=0.0, "Pressure - HI 2"=0.0, "Pressure - Low"=0.0, "Pres_PIN"=0.0, "UE-State(1/0 on off)"=0.0, "LE-State(1/0 on off)"=0.0, "CALC1"=0.0, "CALC2"=0.0, "CALC3"=0.0, "CALC4"=0.0, "CALC5"=0.0, "CALC6 - 10 Point Moving Avg"=0.0, "NA2"=0.0, "NA3"=0.0} ("MW100 Data Cluster Output") w91] -> w18
    tunnel: [w83 w90] -> w34
    tunnel: [w82 w89] -> w12
    tunnel: [w84 w88] -> w22
    frame "PRAT" {
      n15 = call "PRAT Read All MW100 Inputs.vi"("MW100"=w86, "Error In"=w85) -> ("dup VISA session"=w83:refnum<visa-resource-name>, "PowerData"=w84:T12, "error out"=w82:errorcluster)  [unwired: 11 in]
    }
    frame "HEWH", "HEWH RLT", Default {
      n16 = call "HEWH Read All MW100 Inputs.vi"("MW100"=w93, "LV Program"=w87, "Error In"=w92) -> ("MW100 Output"=w90:refnum<visa-resource-name>, "MW100 Data Cluster Output"=w91:T20, "PowerData"=w88:T12, "Error Out"=w89:errorcluster)  [unwired: 8 in, 1 out]
    }
  }
  "MW100 Output" <- w34
  n17 = Merge Errors(w12, w11, w5) -> (w10:errorcluster)
  n18 = case shown="False" w16 {
    tunnel: "Laurel IP Address" -> [_ _]
    tunnel: [w95 w104] -> w23
    tunnel: w22 -> [w101 w102]
    tunnel: [w100 w102] -> w21
    tunnel: [TRUE ("Use Laurel") FALSE ("Use Laurel")] -> w19
    tunnel: w18 -> [w98 w103]
    tunnel: [w97 w103] -> w17
    tunnel: w14 -> [w94 _]
    tunnel: w13 -> [w96 _]
    tunnel: w10 -> [w95 w104]
    frame False {
      n19 = Bundle By Name(cluster=w98, "Flow Rate (Linear Link GPM) - Calculated"=w94, "Totalized Flow (Linear Link GAL) - Calculated"=w96) -> (w97:T20)
      n20 = Bundle By Name(cluster=w101, "HEWH Standard.Flow Rate (GPM)"=w94, "HEWH Standard.Gallons (Gal)"=w96) -> (w100:T12)
    }
    frame True {
    }
  }
  n21 = case shown="\"HEWH\"" w25 {
    tunnel: w23 -> [w107 w116]
    tunnel: [w107 w115] -> w33
    tunnel: "Yokogawa WT210" -> [_ w110]
    tunnel: w21 -> [w106 w114]
    tunnel: [w106 w113] -> w31
    tunnel: w9 -> [_ w112]
    tunnel: w6 -> [_ w108]
    frame "PRAT", "HEWH RLT", Default {
      # "PRAT does not use the WT series power analyzers. They are the standard voltage output \ntranducers. I will get this data after scanning the MW100"
    }
    frame "HEWH" {
      # "It is setup to run either a WT200 or WT300"
      n22 = Equal?(x=refnum<visa-resource-name> refnum, y=w110) -> (x = y?=w109:bool)
      n23 = case shown="\"WT300\"" w112 {
        tunnel: w116 -> [w117 w125 w147]
        tunnel: [w117 w124 w145] -> w115
        tunnel: w110 -> [_ w121 w144]
        tunnel: w114 -> [w118 w123 w148]
        tunnel: [w118 w122 w146] -> w113
        tunnel: w109 -> [_ w120 w149]
        tunnel: w108 -> [_ w119 w143]
        frame Default {
        }
        frame "WT300" {
          n24 = case shown="False" w120 {
            tunnel: w125 -> [w127 w141]
            tunnel: [w127 w141] -> w124
            tunnel: w123 -> [w140 w142]
            tunnel: [w139 w142] -> w122
            tunnel: w121 -> [_ _]
            tunnel: w119 -> [w126 _]
            frame False {
              n25 = Unbundle By Name(w126) -> ("Voltage (V):Element 1"=w138:dbl, "Current (A):Element 1"=w137:dbl, "Power (W):Sigma"=w136:dbl, "Watt Hours (Wh):Sigma"=w135:dbl, "Voltage Harmonic (%):Element 1"=w134:dbl, "Frequency (Hz):Element 1"=w133:dbl, "Apparent Power (VA):Element 1"=w132:dbl, "Power Factor:Element 1"=w131:dbl, "Current Crest Factor:Element 1"=w130:dbl, "Voltage Crest Factor:Element 1"=w129:dbl, "Time:Element 1"=w128:dbl)
              n26 = Bundle By Name(cluster=w140, "HEWH Standard.Voltage (Volts)"=w138, "HEWH Standard.Current (Amps)"=w137, "HEWH Standard.Power (Watts)"=w136, "HEWH Standard.WattHours (Wh)"=w135, "Additional Power Data.Vthd"=w134, "Additional Power Data.Frequency (Hz)"=w133, "Additional Power Data.Apparent Power (VA)"=w132, "Additional Power Data.Power Factor"=w131, "Additional Power Data.Current Crest Factor"=w130, "Additional Power Data.Voltage Crest Factor"=w129, "Additional Power Data.Integration Time (sec)"=w128) -> (w139:T12)
            }
            frame True {
            }
          }
        }
        frame "WT210" {
          n27 = case shown="True" w149 {
            tunnel: w148 -> [w164 w165]
            tunnel: w147 -> [w150 w166]
            tunnel: [w150 w166] -> w145
            tunnel: [w163 w165] -> w146
            tunnel: w144 -> [_ _]
            tunnel: w143 -> [w151 _]
            frame False {
              n28 = Unbundle By Name(w151) -> ("Voltage (V):Element 1"=w162:dbl, "Current (A):Element 1"=w161:dbl, "Power (W):Sigma"=w160:dbl, "Watt Hours (Wh):Sigma"=w159:dbl, "Voltage Harmonic (%):Element 1"=w158:dbl, "Frequency (Hz):Element 1"=w157:dbl, "Apparent Power (VA):Element 1"=w156:dbl, "Power Factor:Element 1"=w155:dbl, "Current Crest Factor:Element 1"=w154:dbl, "Voltage Crest Factor:Element 1"=w153:dbl, "Time:Element 1"=w152:dbl)
              n29 = Bundle By Name(cluster=w164, "HEWH Standard.Voltage (Volts)"=w162, "HEWH Standard.Current (Amps)"=w161, "HEWH Standard.Power (Watts)"=w160, "HEWH Standard.WattHours (Wh)"=w159, "Additional Power Data.Vthd"=w158, "Additional Power Data.Frequency (Hz)"=w157, "Additional Power Data.Apparent Power (VA)"=w156, "Additional Power Data.Power Factor"=w155, "Additional Power Data.Current Crest Factor"=w154, "Additional Power Data.Voltage Crest Factor"=w153, "Additional Power Data.Integration Time (sec)"=w152) -> (w163:T12)
            }
            frame True {
            }
          }
        }
      }
    }
  }
  n30 = call "HEWH Determine Events.vi"("Core HEWH Data in"=w28, "PowerData"=w31, "Error In"=w33, "GEA2?"="GEA2?") -> ("Core HEWH Data out"=w36:T2, "Error Out"=w35:errorcluster)  [unwired: 10 in]
  "Core HEWH Data Station A" <- w36
  n31 = call "HEWH Parse Heatup Test Data.vi"("Emerson Flow Meter Data Input"=w4, "Use Laurel"=w19, "Error In"=w35, "Use Emerson 5700?"="Use Emerson 5700?", "MW100 Data Cluster"=w17, "Core HEWH Data Station In"=w36) -> ("Error Out"=→"error out":errorcluster, "Emerson Flow Meter Data Output"=→"Emerson Flow Meter Data Output":T1, "Output Data"=→"MW100 Full Data":string[][], "Display Message"=→"Display Message":string)  [unwired: 2 in]
